vi "Get Galaxy Pairs.vi"(0 "Galaxy Locations":cdb[](array[numeric])) -> (2 "Galaxy Pairs":set{set{cdb}}(c389))   [LabVIEW 2020, in "AoC 2023.lvlib"]
uses:
  AoC 2023.lvlib
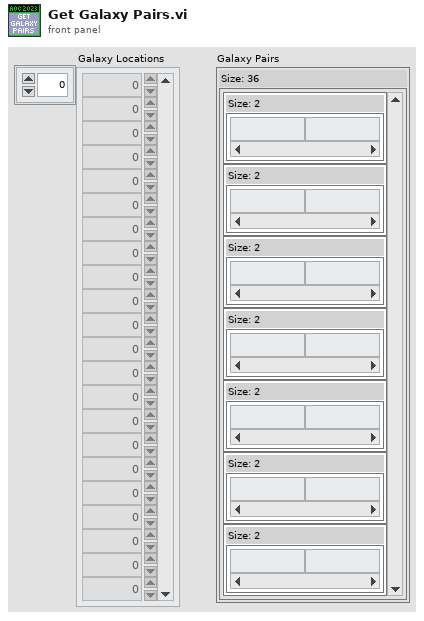
[diagram p1: front panel]
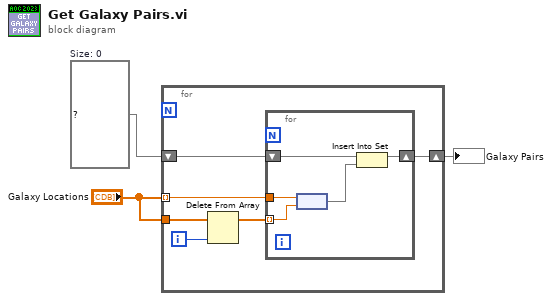
[diagram p0: block diagram]
diagram:
  w3 = set{set{cdb}} {}  # Size: 0
  n1 = for {
    tunnel: "Galaxy Locations" -> [w9] mode=indexing
    tunnel: "Galaxy Locations" -> [w6]
    shift-right: [w8] -> w1
    shift-left: w3 -> [w7]
    i -> [w4]
    n2 = Delete From Array(array=w6, index=w4) -> (array with subset deleted=w5:cdb[])  [unwired: 1 in, 1 out]
    n3 = for {
      tunnel: w9 -> [w14]
      tunnel: w5 -> [w13] mode=indexing
      shift-right: [w11] -> w8
      shift-left: w7 -> [w10]
      n4 = node(w14, w13) -> (w12:set{cdb})
      n5 = Insert Into Set(10:w12, 11:w10) -> (3:w11:set{set{cdb}})  [unwired: 1 out]
    }
  }
  "Galaxy Pairs" <- w1
